vi "KF_sub.vi"(4 "H Matrix":T1, 6 "F  Matrix":T1, 8 "Observations 1 Gyro Velocity":dbl format="%#_13g", 9 "Steady State Kalman Predictor Gain matrix":T1, 10 "Observations 2 Accelerometer ANGLE in degrees":dbl format="%#_13g", 11 "X from register":dbl[](array[numeric])) -> (3 "X^ to register":dbl[](array[numeric]))   [LabVIEW 2016]
uses:
  <vilib>/Analysis/NI_AALBase.lvlib
  <vilib>/Analysis/baseanly.llb/A x Vector.vi
  <vilib>/Analysis/Matrix/Datatypes/RealMatrix.ctl
  <vilib>/Analysis/Matrix/NI_Matrix.lvlib
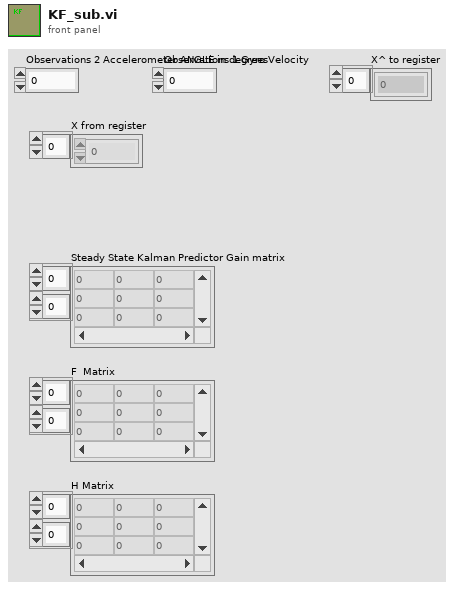
[diagram p1: front panel]
types:
  T1 = typedef "NI_Matrix.lvlib/RealMatrix.ctl" = dbl[][]
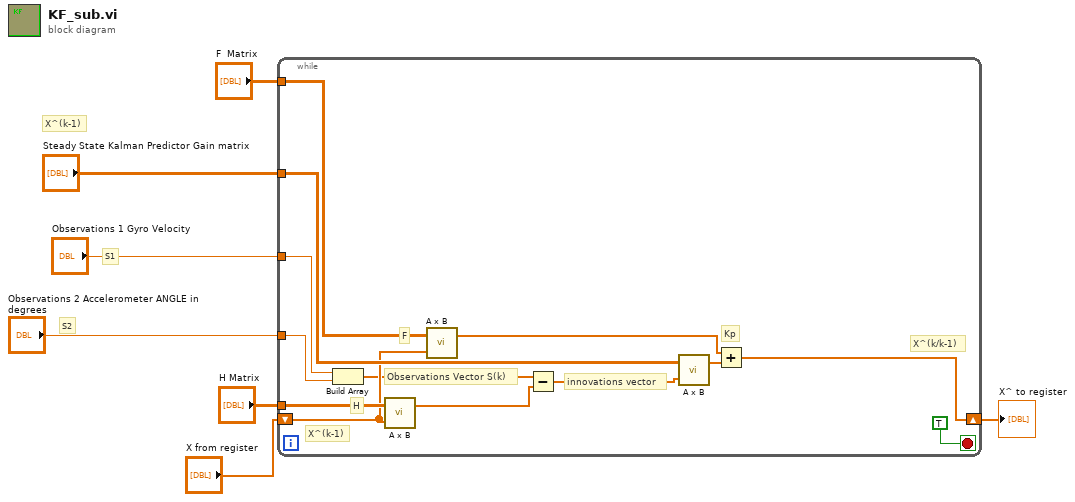
[diagram p0: block diagram]
diagram:
  # "X^(k-1)"
  # "S2"
  # "S1"
  n1 = while {
    tunnel: "Steady State Kalman Predictor Gain matrix" -> [w15]
    tunnel: "F  Matrix" -> [w17]
    tunnel: "H Matrix" -> [w19]
    shift-right: [w18] -> w6
    shift-left: "X from register" -> [w11]
    tunnel: "Observations 1 Gyro Velocity" -> [w10]
    tunnel: "Observations 2 Accelerometer ANGLE in degrees" -> [w9]
    stop <- TRUE stop-if-true
    # "Observations Vector S(k)"
    # "innovations vector"
    # "X^(k/k-1)"
    # "X^(k-1)"
    # "Kp"
    # "H"
    # "F"
    n2 = Build Array(w10, w9) -> (w8:dbl[])
    n3 = call-poly <vilib>:"A x B.vi"("Vector"=w11, "A"=w19) -> ("A x Vector"=w13:dbl[])  [unwired: 1 out]
    n4 = call-poly <vilib>:"A x B.vi"("Vector"=w11, "A"=w17) -> ("A x Vector"=w16:dbl[])  [unwired: 1 out]
    n5 = Subtract(x=w8, y=w13) -> (x-y=w12:dbl[])
    n6 = call-poly <vilib>:"A x B.vi"("Vector"=w12, "A"=w15) -> ("A x Vector"=w14:dbl[])  [unwired: 1 out]
    n7 = Add ("Add.vi")(x=w16, y=w14) -> (x+y=w18:dbl[])
  }
  "X^ to register" <- w6
